vi "Inst.RP100.getAll.vi"(8 "error in (no error)":errorcluster, 11 "Inst.RP100 in":refnum<class "Inst.RP100.lvclass">) -> (0 "error out":errorcluster, 2 "output cluster":T1, 3 "Inst.RP100 out":refnum<class "Inst.RP100.lvclass">)   [LabVIEW 2019, in "Inst.RP100.lvclass"]
uses:
  Inst.RP100.lvclass
  Typedefs/Output Channel--Enum.ctl
  Typedefs/Inst.RP100.getAll--Cluster.ctl
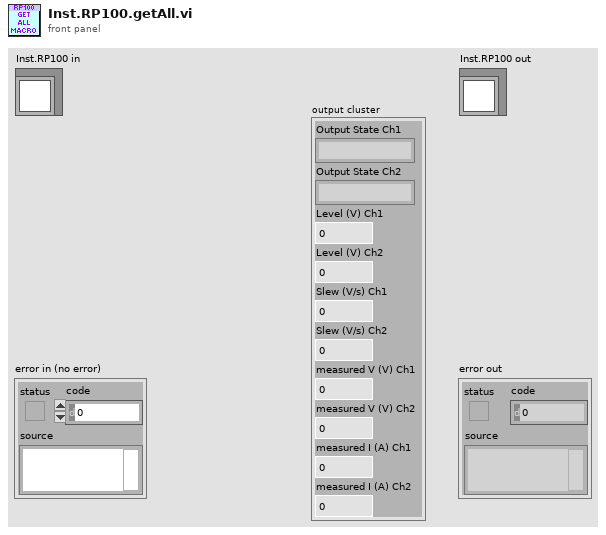
[diagram p1: front panel]
types:
  T1 = typedef "Inst.RP100.lvclass/Inst.RP100.getAll--Cluster.ctl" = cluster{"Output State Ch1":string, "Output State Ch2":string, "Level (V) Ch1":dbl, "Level (V) Ch2":dbl, "Slew (V/s) Ch1":dbl, "Slew (V/s) Ch2":dbl, "measured V (V) Ch1":dbl, "measured V (V) Ch2":dbl, "measured I (A) Ch1":dbl, "measured I (A) Ch2":dbl}
  T2 = typedef "Inst.RP100.lvclass/Output Channel--Enum.ctl" = enum16{"Output 1", "Output 2"}
  T3 = typedef "Inst.RP100.lvclass/Output State--Enum.ctl" = enum16{"Shorted", "Enabled"}
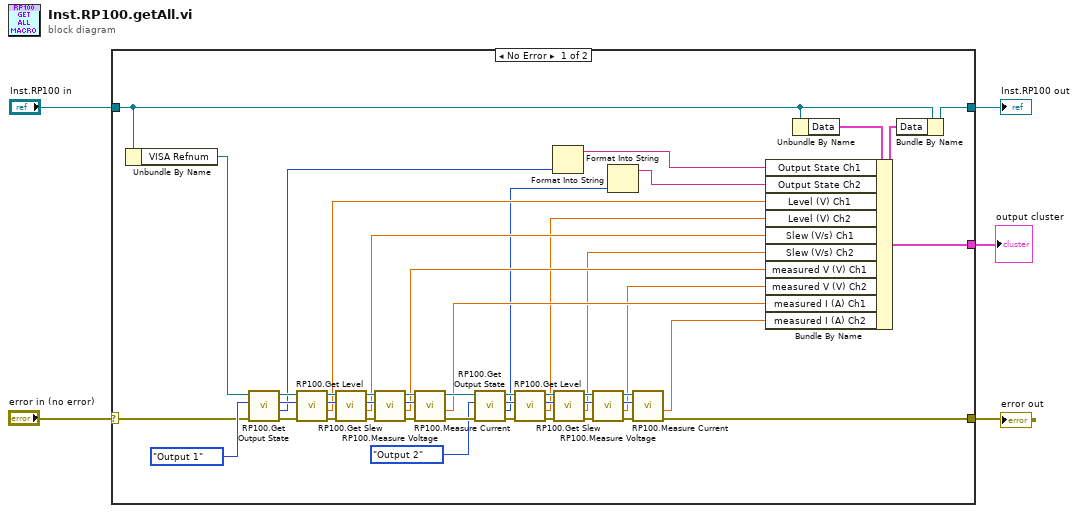
[diagram p0: block diagram]
diagram:
  n1 = case shown="No Error" "error in (no error)" {
    selector: "error in (no error)" -> [w7 w54]
    tunnel: [w10 w54] -> w3
    tunnel: [w15 w53] -> w2
    tunnel: "Inst.RP100 in" -> [w9 w53]
    tunnel: [w6 _] -> w1
    frame No Error {
      n2 = Unbundle By Name(w9) -> ("VISA Refnum"=w8:refnum<visa-resource-name>)
      n3 = call "RP100.Get Output State.vi"("error in (no error)"=w7, "Output Channel"=Output_Channel--Enum."Output 1", "VISA resource name"=w8) -> ("error out"=w41:errorcluster, "Output State"=w14:T3, "Output Channel"=w30:T2, "VISA Refnum out"=w42:refnum<visa-resource-name>)  [unwired: 5 in]
      n4 = call "RP100.Get Level.vi"("error in (no error)"=w41, "Output Channel"=w30, "VISA resource name"=w42) -> ("error out"=w39:errorcluster, "Level (V)"=w24:dbl, "Output Channel"=w29:T2, "VISA Refnum out"=w40:refnum<visa-resource-name>)  [unwired: 5 in]
      n5 = call "RP100.Get Slew.vi"("error in (no error)"=w39, "Output Channel"=w29, "VISA resource name"=w40) -> ("error out"=w37:errorcluster, "Slew (V/s)"=w23:dbl, "Output Channel"=w28:T2, "VISA Refnum out"=w38:refnum<visa-resource-name>)  [unwired: 5 in]
      n6 = call "RP100.Measure Voltage.vi"("error in (no error)"=w37, "Output"=w28, "VISA resource name"=w38) -> ("error out"=w51:errorcluster, "measured V"=w22:dbl, "Output"=w50:T2, "VISA Refnum out"=w52:refnum<visa-resource-name>)  [unwired: 5 in]
      n7 = call "RP100.Measure Current.vi"("error in (no error)"=w51, "Output Channel"=w50, "VISA resource name"=w52) -> ("error out"=w46:errorcluster, "measured I"=w21:dbl, "VISA Refnum out"=w45:refnum<visa-resource-name>)  [unwired: 5 in, 1 out]
      n8 = call "RP100.Get Output State.vi"("error in (no error)"=w46, "Output Channel"=Output_Channel--Enum."Output 2", "VISA resource name"=w45) -> ("error out"=w35:errorcluster, "Output State"=w12:T3, "Output Channel"=w27:T2, "VISA Refnum out"=w36:refnum<visa-resource-name>)  [unwired: 5 in]
      n9 = call "RP100.Get Level.vi"("error in (no error)"=w35, "Output Channel"=w27, "VISA resource name"=w36) -> ("error out"=w33:errorcluster, "Level (V)"=w20:dbl, "Output Channel"=w26:T2, "VISA Refnum out"=w34:refnum<visa-resource-name>)  [unwired: 5 in]
      n10 = Format Into String(w14) -> (resulting string=w13:string)  [unwired: 3 in, 1 out]
      n11 = call "RP100.Get Slew.vi"("error in (no error)"=w33, "Output Channel"=w26, "VISA resource name"=w34) -> ("error out"=w31:errorcluster, "Slew (V/s)"=w19:dbl, "Output Channel"=w25:T2, "VISA Refnum out"=w32:refnum<visa-resource-name>)  [unwired: 5 in]
      n12 = call "RP100.Measure Voltage.vi"("error in (no error)"=w31, "Output"=w25, "VISA resource name"=w32) -> ("error out"=w48:errorcluster, "measured V"=w18:dbl, "Output"=w49:T2, "VISA Refnum out"=w47:refnum<visa-resource-name>)  [unwired: 5 in]
      n13 = Format Into String(w12) -> (resulting string=w11:string)  [unwired: 3 in, 1 out]
      n14 = call "RP100.Measure Current.vi"("error in (no error)"=w48, "Output Channel"=w49, "VISA resource name"=w47) -> ("error out"=w10:errorcluster, "measured I"=w17:dbl)  [unwired: 5 in, 2 out]
      n15 = Unbundle By Name(w9) -> ("Data"=w16:T1)
      n16 = Bundle By Name(cluster=w16, "Output State Ch1"=w13, "Output State Ch2"=w11, "Level (V) Ch1"=w24, "Level (V) Ch2"=w20, "Slew (V/s) Ch1"=w23, "Slew (V/s) Ch2"=w19, "measured V (V) Ch1"=w22, "measured V (V) Ch2"=w18, "measured I (A) Ch1"=w21, "measured I (A) Ch2"=w17) -> (w6:T1)
      n17 = Bundle By Name(cluster=w9, "Data"=w6) -> (w15:refnum<class "Inst.RP100.lvclass">)
    }
    frame Error {
    }
  }
  "error out" <- w3
  "Inst.RP100 out" <- w2
  "output cluster" <- w1
